vi "Reply.vi"(7 "Sender":refnum<class "Sender.lvclass">, 9 "Priority?":bool, 10 "Msg Strategy":refnum<class "Msg Strategy.lvclass">, 11 "Base jettl in":refnum<class "Base jettl.lvclass">) -> (3 "Base jettl out":refnum<class "Base jettl.lvclass">)   [LabVIEW 2021, in "jettl.lvlib" / "Base jettl.lvclass"]
uses:
  Base jettl.lvclass
  Sender/Sender/Sender.lvclass
  Msg Strategy/Msg Strategy.lvclass
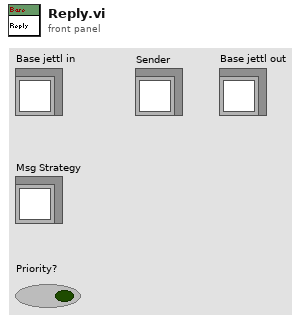
[diagram p1: front panel]
types:
  T1 = typedef "jettl.lvlib/Sender.lvlib/Relation.ctl" = enum16{"Self", "Creator", "Created"}
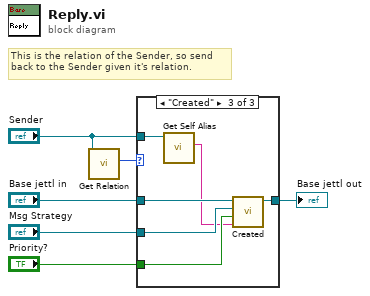
[diagram p0: block diagram]
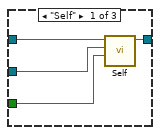
[diagram p2: hidden frame]
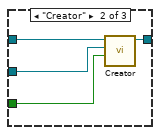
[diagram p3: hidden frame]
diagram:
  # "This is the relation of the Sender, so send back to the Sender given it's relation."
  n1 = call-dynamic "Get Relation.vi"("Sender in"="Sender") -> ("Relation"=w6:T1)  [unwired: 10 in]
  n2 = case shown="\"Created\"" w6 {
    tunnel: [w9 w13 w19] -> w5
    tunnel: "Base jettl in" -> [w10 w14 w20]
    tunnel: "Msg Strategy" -> [w8 w12 w18]
    tunnel: "Priority?" -> [w7 w11 w17]
    tunnel: "Sender" -> [_ _ w16]
    frame "Self" {
      n3 = call-dynamic "Self.vi"("Priority?"=w7, "Msg Strategy"=w8, "Base jettl in"=w10) -> ("Base jettl out"=w9:refnum<class "Base jettl.lvclass">)  [unwired: 8 in]
    }
    frame "Creator" {
      n4 = call-dynamic "Creator.vi"("Priority?"=w11, "Msg Strategy"=w12, "Base jettl in"=w14) -> ("Base jettl out"=w13:refnum<class "Base jettl.lvclass">)  [unwired: 8 in]
    }
    frame "Created" {
      n5 = call-dynamic "Get Self Alias.vi"("Sender in"=w16) -> ("Self Alias"=w15:string)  [unwired: 10 in]
      n6 = call-dynamic "Created.vi"("Created Alias"=w15, "Priority?"=w17, "Msg Strategy"=w18, "Base jettl in"=w20) -> ("Base jettl out"=w19:refnum<class "Base jettl.lvclass">)  [unwired: 7 in]
    }
  }
  "Base jettl out" <- w5
